vi "Shi move.vi"(1 "Color":i32, 2 "Array Position":cluster{"Row":i32, "Column":i32}, 3 "Chess Array":i32[][](array[numeric])=[[140, 130, 120, 110, 100, 111, 121, 131, 141], [-1, -1, -1, -1, -1, -1, -1, -1, -1], [-1, 150, -1, -1, -1, -1, -1, 151, -1], [160, -1, 161, -1, 162, -1, 163, -1, 164], [-1, -1, -1, -1, -1, -1, -1, -1, -1], [-1, -1, -1, -1, -1, -1, -1, -1, -1], [260, -1, 261, -1, 262, -1, 263, -1, 264], [-1, 250, -1, -1, -1, -1, -1, 251, -1], [-1, -1, -1, -1, -1, -1, -1, -1, -1], [240, 230, 220, 210, 200, 211, 221, 231, 241]]) -> (0 "Shi move":cluster{i32, i32}[](array[cluster]))   [LabVIEW 2009]
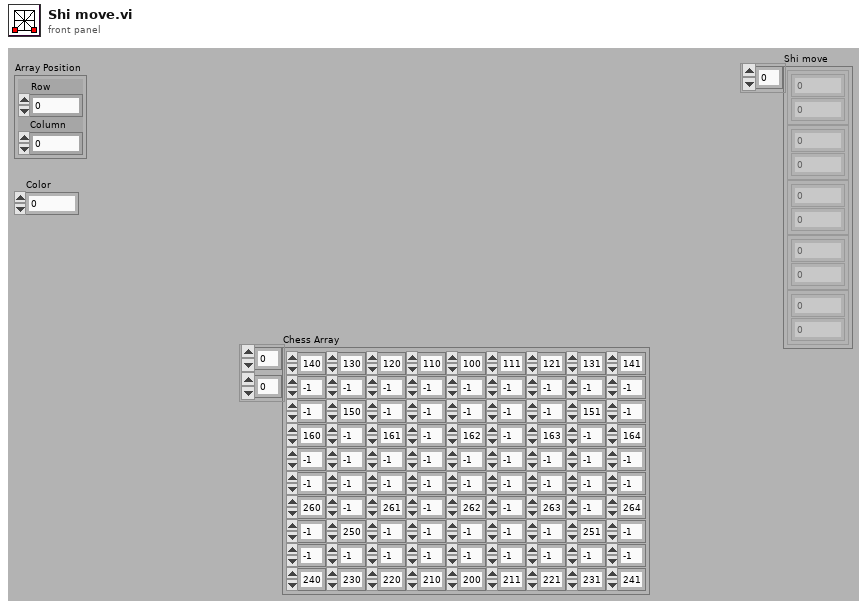
[diagram p1: front panel]
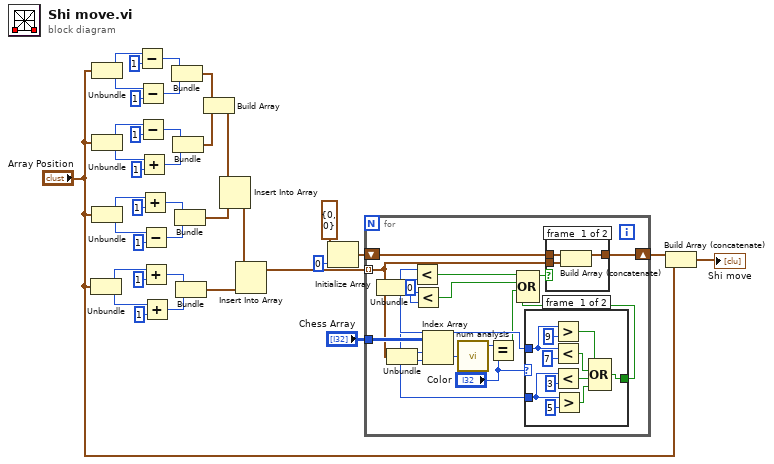
[diagram p0: block diagram]
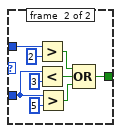
[diagram p2: hidden frame]
diagram:
  n1 = Unbundle("Array Position") -> ("Row"=w30:i32, "Column"=w33:i32)
  n2 = Unbundle("Array Position") -> ("Row"=w38:i32, "Column"=w36:i32)
  n3 = Unbundle("Array Position") -> ("Row"=w35:i32, "Column"=w32:i32)
  n4 = Unbundle("Array Position") -> ("Row"=w31:i32, "Column"=w34:i32)
  n5 = Subtract(x=w38, y=1) -> (x-y=w16:i32)
  n6 = Subtract(x=w36, y=1) -> (x-y=w18:i32)
  n7 = Subtract(x=w35, y=1) -> (x-y=w12:i32)
  n8 = Add(x=w32, y=1) -> (x+y=w14:i32)
  n9 = Add(x=w31, y=1) -> (x+y=w9:i32)
  n10 = Subtract(x=w34, y=1) -> (x-y=w8:i32)
  n11 = Add(x=w30, y=1) -> (x+y=w5:i32)
  n12 = Add(x=w33, y=1) -> (x+y=w4:i32)
  n13 = Bundle(w16, w18) -> (w25:cluster{i32, i32})  [unwired: 1 out]
  n14 = Bundle(w12, w14) -> (w24:cluster{i32, i32})  [unwired: 1 out]
  n15 = Bundle(w9, w8) -> (w22:cluster{i32, i32})  [unwired: 1 out]
  n16 = Bundle(w5, w4) -> (w20:cluster{i32, i32})  [unwired: 1 out]
  n17 = Build Array(w25, w24) -> (w23:cluster{i32, i32}[])
  n18 = Insert Into Array(array=w23, new element=w22) -> (w21:cluster{i32, i32}[])  [unwired: 1 in]
  n19 = Insert Into Array(array=w21, new element=w20) -> (w29:cluster{i32, i32}[])  [unwired: 1 in]
  n20 = Initialize Array(cluster{i32, i32} {0, 0} ("Output Cluster"), 0 ("Dimension Size")) -> (w28:cluster{i32, i32}[])
  n21 = for {
    tunnel: w29 -> [w44] mode=indexing
    shift-right: [w50] -> w3
    shift-left: w28 -> [w51]
    tunnel: "Chess Array" -> [w49]
    w55 = 0 ("y")
    n22 = Unbundle(w44) -> (w43:i32, w39:i32)
    n23 = Unbundle(w44) -> (w46:i32, w45:i32)
    n24 = Less?(x=w43, y=w55) -> (x < y?=w53:bool)
    n25 = Less?(x=w39, y=w55) -> (x < y?=w54:bool)
    n26 = Index Array(array=w49, index (row)=w46, index (col)=w45) -> (element=w48:i32)
    n27 = call "num analysis.vi"("x"=w48) -> ("Color"=w47:i32)  [unwired: 2 out]
    n28 = Equal?(x=w47, y="Color") -> (x = y?=w41:bool)
    n29 = case shown="1, Default" "Color" {
      tunnel: w43 -> [w58 w74]
      tunnel: w39 -> [w64 w71]
      tunnel: [w66 w75] -> w40
      frame #0 {
        n30 = Greater?(x=w58, y=9) -> (0:w56:bool)
        n31 = Less?(x=w58, y=7) -> (x < y?=w62:bool)
        n32 = Less?(x=w64, y=3) -> (x < y?=w61:bool)
        n33 = Greater?(x=w64, y=5) -> (0:w60:bool)
        n34 = Compound Arithmetic op=OR(w56, w62, w61, w60) -> (w66:bool)
      }
      frame #1 {
        n35 = Greater?(x=w74, y=2) -> (0:w69:bool)
        n36 = Less?(x=w71, y=3) -> (x < y?=w68:bool)
        n37 = Greater?(x=w71, y=5) -> (0:w67:bool)
        n38 = Compound Arithmetic op=OR(w69, w68, w67) -> (w75:bool)
      }
    }
    n39 = Compound Arithmetic op=OR(w53, w54, w41, w40) -> (w52:bool)
    n40 = case shown="False" w52 {
      tunnel: w51 -> [w78 w79]
      tunnel: [w77 w79] -> w50
      tunnel: w44 -> [w76 _]
      frame #0 {
        n41 = Build Array (concatenate)(w78, w76) -> (w77:cluster{i32, i32}[])
      }
      frame #1 {
      }
    }
  }
  n42 = Build Array (concatenate)(w3, "Array Position") -> (→"Shi move":cluster{"Row":i32, "Column":i32}[])
